vi "Open Command Panel.vi"(10 "Commands":cluster{"Time (s)":dbl, T1, bool}[](array[cluster]), 11 "Tag":string) -> (3 "Found":bool)   [LabVIEW 2019]
uses:
  Single Cmd Info.ctl
  <vilib>/picture/picture.llb/imagedata.ctl
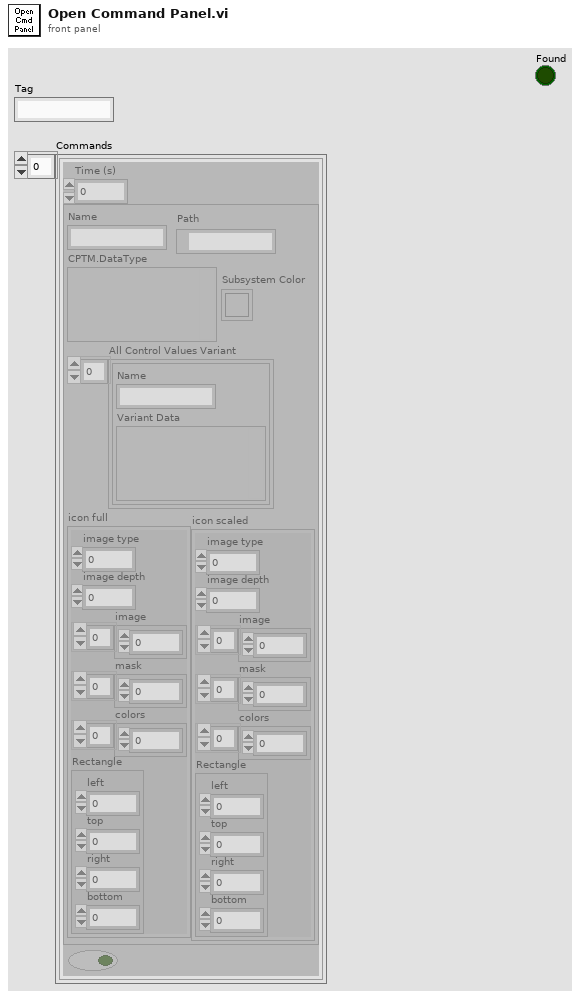
[diagram p1: front panel]
types:
  T1 = typedef "Single Cmd Info.ctl" = cluster{"Name":string, "CPTM.DataType":variant, "All Control Values Variant":cluster{"Name":string, "Variant Data":variant}[], "icon full":T2, "icon scaled":T2, "Path":path, "Subsystem Color":u32}
  T2 = typedef "imagedata.ctl" = cluster{"image type":i32, "image depth":i32, "image":u8[], "mask":u8[], "colors":u32[], "Rectangle":cluster{"left":i16, "top":i16, "right":i16, "bottom":i16}}
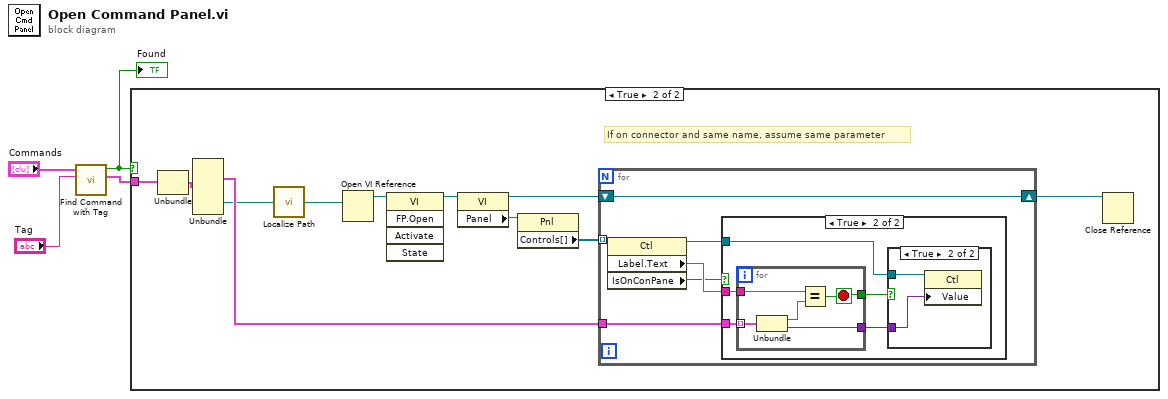
[diagram p0: block diagram]
diagram:
  n1 = call "Find Command with Tag.vi"("Command Tag"="Tag", "Commands"="Commands") -> ("Found Command"=w3:cluster{"Time (s)":dbl, T1, bool}, "Found"=w2:bool)  [unwired: 7 in, 1 out]
  "Found" <- w2
  n2 = case shown="True" w2 {
    tunnel: w3 -> [_ w14]
    frame False {
    }
    frame True {
      # "If on connector and same name, assume same parameter"
      n3 = Unbundle(w14) -> (w13:T1)  [unwired: 2 out]
      n4 = Unbundle(w13) -> ("All Control Values Variant"=w9:cluster{"Name":string, "Variant Data":variant}[], "Path"=w6:path)  [unwired: 5 out]
      n5 = call "Localize Path.vi"("Path"=w6) -> ("Local path"=w5:path)
      n6 = Open VI Reference(vi path=w5) -> (vi reference=w15:refnum<vi>)  [unwired: 5 in, 1 out]
      n7 = invoke class="VI" method="FP.Open"(reference=w15) -> (reference out=w11:refnum<vi>)  [unwired: 4 in, 4 out]
      n8 = property class="VI"(reference=w11) -> (reference out=w8:refnum<vi>, "Panel"=w12:refnum<vi>)  [unwired: 1 in, 1 out]
      n9 = property class="Pnl"(reference=w12) -> ("Controls[]"=w10:refnum<vi>[])  [unwired: 1 in, 2 out]
      n10 = for {
        tunnel: w10 -> [w20] mode=indexing
        tunnel: w9 -> [w21]
        shift-right: [w16] -> w7
        shift-left: w8 -> [w16]
        n11 = property class="Ctl"(reference=w20) -> (reference out=w17:refnum<vi>, "Label.Text"=w19:string, "IsOnConPane"=w18:bool)  [unwired: 1 in, 1 out]
        n12 = case shown="True" w18 {
          tunnel: w21 -> [_ w26]
          tunnel: w19 -> [_ w25]
          tunnel: w17 -> [_ w24]
          frame False {
          }
          frame True {
            n13 = for {
              tunnel: w26 -> [w33] mode=indexing
              tunnel: [w32] -> w23
              tunnel: w25 -> [w31]
              tunnel: [w29] -> w22
              stop <- w29 stop-if-true
              n14 = Unbundle(w33) -> ("Name"=w30:string, "Variant Data"=w32:variant)
              n15 = Equal?(x=w31, y=w30) -> (x = y?=w29:bool)
            }
            n16 = case shown="True" w22 {
              tunnel: w24 -> [_ w28]
              tunnel: w23 -> [_ w27]
              frame False {
              }
              frame True {
                n17 = property class="Ctl"(reference=w28, "Value"=w27) -> ()  [unwired: 1 in, 2 out]
              }
            }
          }
        }
      }
      n18 = Close Reference(reference=w7) -> ()  [unwired: 1 in, 1 out]
    }
  }
